vi "FGV Messwerte zusammenfassen.vi"(6 "Aktionen":T1, 7 "labBaseName":string, 8 "LabBaseNr":i32, 9 "FTIR Status":sgl[](array[numeric]), 10 "Algebraic":sgl[](array[numeric]), 11 "FT-IR":sgl[](array[numeric])) -> (0 "LabBaseNr":i32, 1 "FTIR Status":sgl[](array[numeric]), 2 "Algebraic":sgl[](array[numeric]), 3 "FT-IR":sgl[](array[numeric]), 5 "labBaseName":string)   [LabVIEW 2020, in "Messdaten.lvlib"]
uses:
  Messdaten.lvlib
  Aktionen FGV Messwerte zusammenfassen.ctl
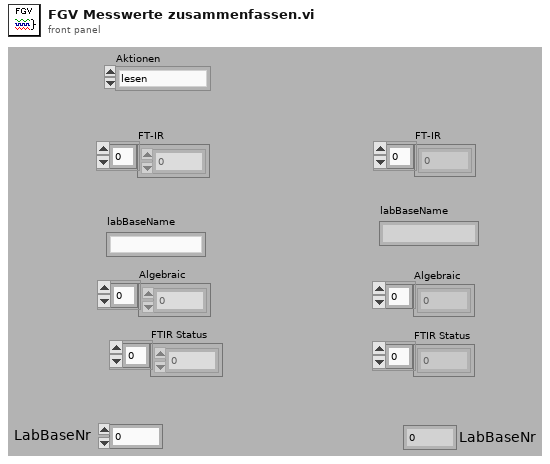
[diagram p1: front panel]
types:
  T1 = typedef "Messdaten.lvlib/Aktionen FGV Messwerte zusammenfassen.ctl" = enum16{"lesen", "FT-IR", "Algebraic", "LabBaseName", "LabBaseNr"}
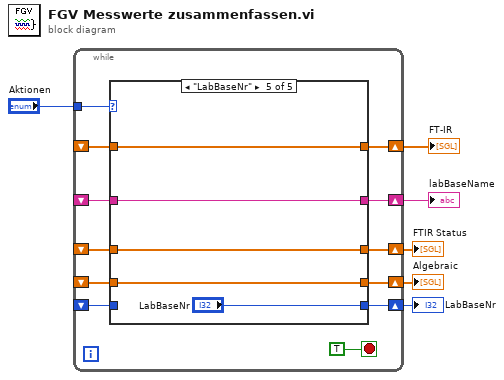
[diagram p0: block diagram]
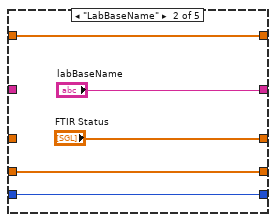
[diagram p3: hidden frame]
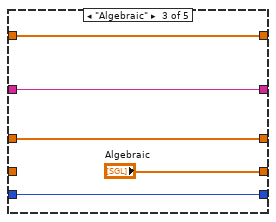
[diagram p4: hidden frame]
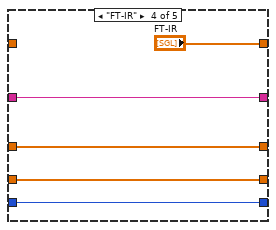
[diagram p5: hidden frame]
diagram:
  n1 = while {
    tunnel: "Aktionen" -> [w18]
    shift-right: [w16] -> w4
    shift-left: _ -> [w14]
    shift-right: [w15] -> w5
    shift-left: _ -> [w13]
    shift-right: [w12] -> w3
    shift-left: _ -> [w11]
    shift-right: [w10] -> w2
    shift-left: _ -> [w9]
    shift-right: [w8] -> w1
    shift-left: _ -> [w7]
    stop <- TRUE stop-if-true
    n2 = case shown="\"LabBaseNr\"" w18 {
      tunnel: [w23 w28 w33 "FT-IR" w40] -> w16
      tunnel: [w22 "labBaseName" w32 w36 w41] -> w15
      tunnel: w14 -> [w23 w28 w33 _ w40]
      tunnel: w13 -> [w22 _ w32 w36 w41]
      tunnel: [w21 w27 "Algebraic" w37 w43] -> w12
      tunnel: w11 -> [w21 w27 _ w37 w43]
      tunnel: [w20 "FTIR Status" w30 w35 w42] -> w10
      tunnel: w9 -> [w20 _ w30 w35 w42]
      tunnel: [w19 w24 w29 w34 "LabBaseNr"] -> w8
      tunnel: w7 -> [w19 w24 w29 w34 _]
      frame "lesen", Default {
      }
      frame "LabBaseName" {
      }
      frame "Algebraic" {
      }
      frame "FT-IR" {
      }
      frame "LabBaseNr" {
      }
    }
  }
  "labBaseName" <- w5
  "FT-IR" <- w4
  "Algebraic" <- w3
  "FTIR Status" <- w2
  "LabBaseNr" <- w1
